vi "Get video data (SubVI).vi"(8 "error in (no error)":errorcluster, 10 "AR Drone Resource":T1, 11 "Numeric":i32) -> (0 "error out":errorcluster, 3 "ImgData":u8[](array[numeric]))   [LabVIEW 2014]
uses:
  <vilib>/LVH/AR Drone Toolkit/Type Defs/AR Drone Resource.ctl
  Drone Project/AR Drone Toolkit (BETA)/Decode Video/2.0/Decode20Video.dll
  <vilib>/LVH/AR Drone Toolkit/AR Drone.lvlib
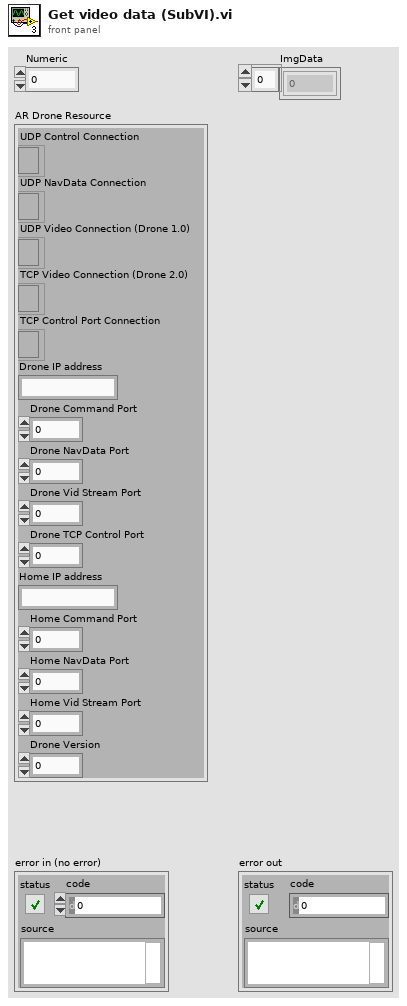
[diagram p1: front panel]
types:
  T1 = typedef "AR Drone.lvlib/AR Drone Resource.ctl" = cluster{"UDP Control Connection":refnum<k16>, "UDP NavData Connection":refnum<k16>, "UDP Video Connection (Drone 1.0)":refnum<k16>, "TCP Video Connection (Drone 2.0)":refnum<k5>, "TCP Control Port Connection":refnum<k5>, "Drone IP address":string, "Drone Command Port":u16, "Drone NavData Port":u16, "Drone Vid Stream Port":u16, "Drone TCP Control Port":u16, "Home IP address":string, "Home Command Port":u16, "Home NavData Port":u16, "Home Vid Stream Port":u16, "Drone Version":i32}
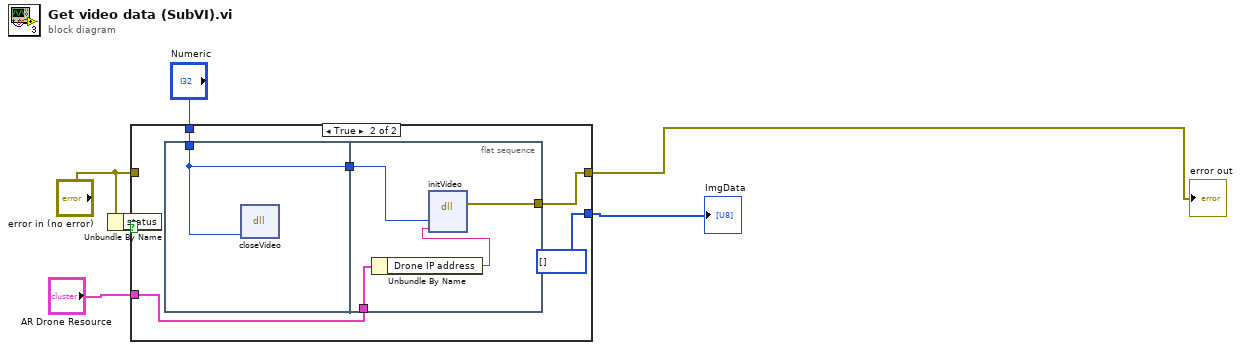
[diagram p0: block diagram]
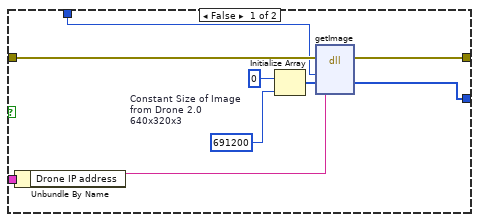
[diagram p2: hidden frame]
diagram:
  n1 = Unbundle By Name("error in (no error)") -> ("status"=w5:bool)
  n2 = case shown="True" w5 {
    tunnel: "error in (no error)" -> [w12 _]
    tunnel: [w8 u8[] [] ("ImgData")] -> w1
    tunnel: "AR Drone Resource" -> [w11 w18]
    tunnel: [w9 w19] -> w3
    tunnel: "Numeric" -> [w7 w20]
    frame False {
      w15 = 691200  # Constant Size of Image from Drone 2.0 640x320x3
      n3 = Unbundle By Name(w11) -> ("Drone IP address"=w10:string)
      n4 = Initialize Array(u8 0 ("dimension size"), w15) -> (w13:u8[])
      n5 = dll-call lib="E:/Dropbox/UTCN/Summer 2015/Drone Project/AR Drone Toolkit (BETA)/Decode Video/2.0/Decode20Video.dll" fn="getImage"(error in=w12, "Index"=w7, "ImgData"=w13, "IP Address"=w10) -> (error out=w9:errorcluster, "ImgData"=w8:u8[])  [unwired: 5 in, 1 out]
    }
    frame True {
      n6 = flat-sequence {
        tunnel: w20 -> [w21]
        tunnel: [w21] -> w17
        tunnel: [w25] -> w19
        tunnel: w18 -> [w24]
        tunnel: w17 -> [w22]
        frame #0 {
          n7 = dll-call lib="E:/Dropbox/UTCN/Summer 2015/Drone Project/AR Drone Toolkit (BETA)/Decode Video/2.0/Decode20Video.dll" fn="closeVideo"("Index"=w21) -> ()  [unwired: 5 in, 2 out]
        }
        frame #1 {
          n8 = Unbundle By Name(w24) -> ("Drone IP address"=w23:string)
          n9 = dll-call lib="E:/Dropbox/UTCN/Summer 2015/Drone Project/AR Drone Toolkit (BETA)/Decode Video/2.0/Decode20Video.dll" fn="initVideo"("Index"=w22, "IP Address"=w23) -> (error out=w25:errorcluster)  [unwired: 6 in, 1 out]
        }
      }
    }
  }
  "error out" <- w3
  "ImgData" <- w1
